vi "Close.vi"(8 "error in":errorcluster, 11 "Power Limit in":refnum<class "Power Limit.lvclass">) -> (0 "error out":errorcluster, 3 "Power Limit out":refnum<class "Power Limit.lvclass">)   [LabVIEW 2023, in "Power Limit.lvclass"]
uses:
  Power Limit.lvclass
  Parents/Limit/Limit.lvclass
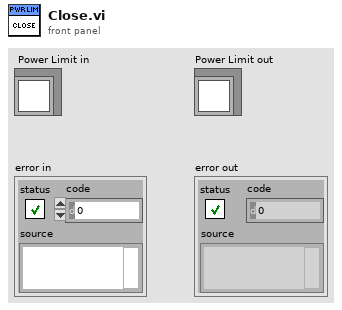
[diagram p1: front panel]
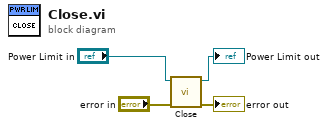
[diagram p0: block diagram]
diagram:
  n1 = call-parent "Close.vi"("error in"="error in", "Limit in"="Power Limit in") -> ("error out"=→"error out":errorcluster, "Limit out"=→"Power Limit out":refnum<class "Power Limit.lvclass">)  [unwired: 8 in]
